vi "genGrooveV3.vi"() -> ()   [LabVIEW 2016]
uses:
  <vilib>/Math Plots/3D Math Plots/3D Scatter/3D Scatter XCtrl/3D Scatter.xctl
  <vilib>/Analysis/1siggen.llb/Ramp Pattern by Samples.vi
  Subsystems/Global Variables.vi
  <vilib>/Math Plots/3D Math Plots/3D Scatter/3D Scatter Datatype/Public/Plot Helper (Vector).vi
  <vilib>/Math Plots/3D Math Plots/3D Scatter/3D Scatter Datatype/3D Scatter Datatype.lvclass
  <vilib>/gmath/NI_Gmath.lvlib
  <vilib>/Analysis/NI_AALBase.lvlib
panel:
  in  "offsetZ":dbl
  in  "offsetX":dbl
  in  "offsetY":dbl
  out "size(s)":i32
  out "zVisTraj":dbl[](array[numeric]) format="%_6g"
  out "yVisTraj":dbl[](array[numeric]) format="%_6g"
  out "xVisTraj":dbl[](array[numeric]) format="%_6g"
  out "Groove Plot":refnum<class "3D Plot Datatype.lvclass">[](xcontrol)
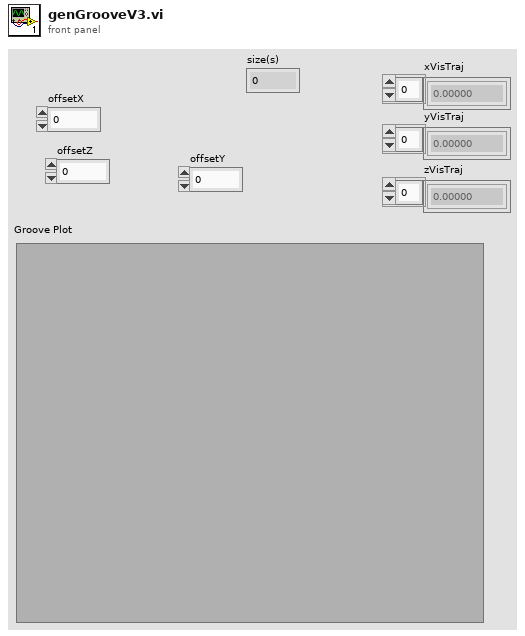
[diagram p1: front panel]
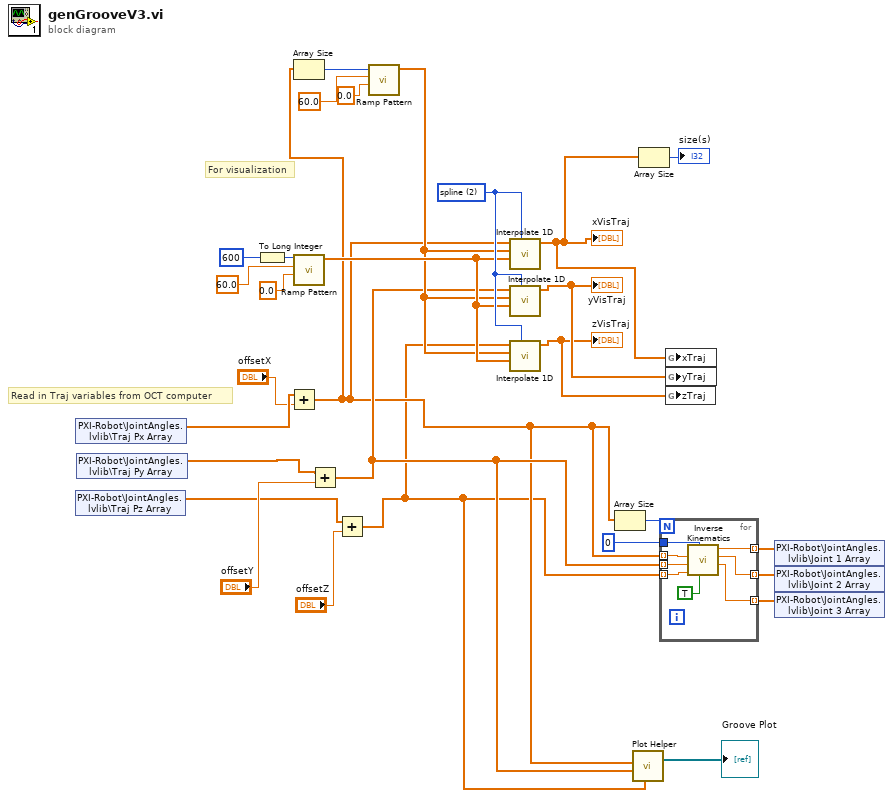
[diagram p0: block diagram]
diagram:
  w29 = 2 items=["nearest", "linear", "spline", "cubic Hermite", "Lagrange"] ("method")
  # "Read in Traj variables from OCT computer"
  # "For visualization"
  n1 = shared-variable "PXI-Robot\\JointAngles.lvlib\\Traj Px Array"() -> (w6:dbl[])  [unwired: 1 in, 1 out]
  n2 = shared-variable "PXI-Robot\\JointAngles.lvlib\\Traj Pz Array"() -> (w3:dbl[])  [unwired: 1 in, 1 out]
  n3 = shared-variable "PXI-Robot\\JointAngles.lvlib\\Traj Py Array"() -> (w9:dbl[])  [unwired: 1 in, 1 out]
  n4 = To Long Integer(number=600) -> (32bit integer=w28:i32)
  n5 = Add(x=w6, y="offsetX") -> (x+y=w5:dbl[])
  n6 = Array Size(array=w5) -> (size(s)=w22:i32)
  n7 = call-poly <vilib>:"Ramp Pattern.vi"("start"=0.0, "end"=60.0, "samples"=w28) -> ("Ramp Pattern"=w26:dbl[])  [unwired: 7 in, 1 out]
  n8 = Add(x=w9, y="offsetY") -> (x+y=w8:dbl[])
  n9 = Add(x=w3, y="offsetZ") -> (x+y=w2:dbl[])
  n10 = call-poly <vilib>:"Ramp Pattern.vi"("start"=0.0, "end"=60.0, "samples"=w22) -> ("Ramp Pattern"=w21:dbl[])  [unwired: 7 in, 1 out]
  n11 = call <vilib>:"Interpolate 1D.vi"("method"=w29, "xi"=w26, "X"=w21, "Y"=w5) -> ("yi"=w18:dbl[])  [unwired: 5 in, 2 out]
  "xVisTraj" <- w18
  n12 = call <vilib>:"Interpolate 1D.vi"("method"=w29, "xi"=w26, "X"=w21, "Y"=w8) -> ("yi"=w17:dbl[])  [unwired: 5 in, 2 out]
  "yVisTraj" <- w17
  n13 = call <vilib>:"Interpolate 1D.vi"("method"=w29, "xi"=w26, "X"=w21, "Y"=w2) -> ("yi"=w16:dbl[])  [unwired: 5 in, 2 out]
  "zVisTraj" <- w16
  n14 = Array Size(array=w5) -> (size(s)=w15:i32)
  n15 = call-poly <vilib>:"Plot Helper.vi"("z vector"=w2, "y vector"=w8, "x vector"=w5) -> ("3D Plot lvclass Array out"=→"Groove Plot":refnum<class "3D Plot Datatype.lvclass">[])  [unwired: 3 in, 5 out]
  n16 = Array Size(array=w18) -> (size(s)=→"size(s)":i32)
  n17 = for {
    N: w15 -> [_]
    tunnel: 0 ("Arm ID Ind") -> [w33]
    tunnel: w5 -> [w37] mode=indexing
    tunnel: w8 -> [w36] mode=indexing
    tunnel: w2 -> [w35] mode=indexing
    tunnel: [w32] -> w14 mode=indexing
    tunnel: [w31] -> w13 mode=indexing
    tunnel: [w30] -> w12 mode=indexing
    n18 = call "Inverse Kinematics.vi"("isToolTipInsideEye"=TRUE, "armID"=w33, "z"=w35, "y"=w36, "x"=w37) -> ("j3"=w30:dbl, "j2"=w31:dbl, "j1"=w32:dbl)  [unwired: 3 in, 1 out]
  }
  n19 = global write "Global Variables.vi" "xTraj"(w18) -> ()
  n20 = global write "Global Variables.vi" "yTraj"(w17) -> ()
  n21 = global write "Global Variables.vi" "zTraj"(w16) -> ()
  n22 = shared-variable "PXI-Robot\\JointAngles.lvlib\\Joint 1 Array"(w14) -> ()  [unwired: 1 in, 1 out]
  n23 = shared-variable "PXI-Robot\\JointAngles.lvlib\\Joint 2 Array"(w13) -> ()  [unwired: 1 in, 1 out]
  n24 = shared-variable "PXI-Robot\\JointAngles.lvlib\\Joint 3 Array"(w12) -> ()  [unwired: 1 in, 1 out]
